vi "SSL Detection Frame Balls Estimator - Copia.vi"(5 "Time Stamp":timestamp, 7 "Life Time":dbl=1.0) -> ()   [LabVIEW 2016]
uses:
  SSL Detection Robot.ctl
panel:
  out "Est. Robots":T1[](array[typedef]) {"height" format="%+4.3f"; "pixel_y" format="%+4.3f"; "pixel_x" format="%+4.3f"; "orientation" format="%+4.3f"; "y" format="%+4.3f"; "confidence" format="%4.3f"; "x" format="%+4.3f"}
  in  "Robots":T1[](array[typedef]) {"height" format="%+4.3f"; "pixel_y" format="%+4.3f"; "pixel_x" format="%+4.3f"; "orientation" format="%+4.3f"; "y" format="%+4.3f"; "confidence" format="%4.3f"; "x" format="%+4.3f"}
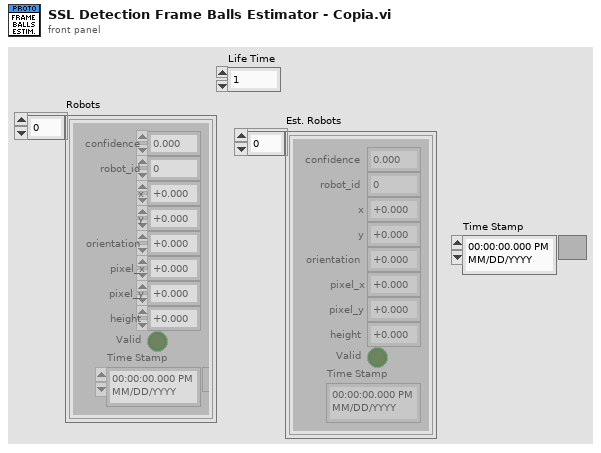
[diagram p1: front panel]
types:
  T1 = typedef "SSL Detection Robot.ctl" = cluster{"x":dbl, "robot_id":u32, "confidence":sgl, "y":sgl, "orientation":sgl, "pixel_x":sgl, "pixel_y":sgl, "height":sgl, "Valid":bool, "Time Stamp":timestamp}
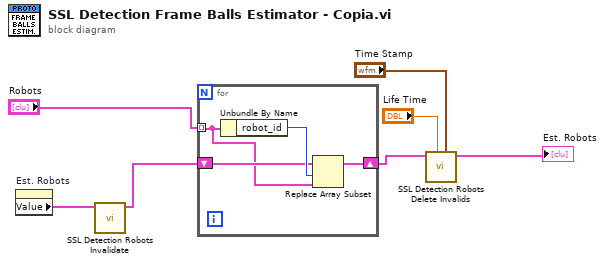
[diagram p0: block diagram]
diagram:
  n1 = property on="Est. Robots" class="Arr (strict)"() -> ("Value"=w5:T1[])  [unwired: 2 in, 2 out]
  n2 = call "SSL Detection Robots Invalidate.vi"("Value"=w5) -> ("Array"=w3:T1[])  [unwired: 10 in]
  n3 = for {
    tunnel: "Robots" -> [w8] mode=indexing
    shift-right: [w9] -> w2
    shift-left: w3 -> [w10]
    n4 = Unbundle By Name(w8) -> ("robot_id"=w11:u32)
    n5 = Replace Array Subset(array=w10, new element=w8, index=w11) -> (w9:T1[])
  }
  n6 = call "SSL Detection Robots Delete Invalids.vi"("Now"="Time Stamp", "Life Time"="Life Time", "Robots In"=w2) -> ("Robots Out"=→"Est. Robots":T1[])  [unwired: 8 in]
